vi "LabVIEW Verifier VI.vi"() -> ()   [LabVIEW 2020]
panel:
  out "Stabilization":u16(slide) scale=0.0..500.0
  out "Overall Verification":bool
  in  "Test Points & Results":T1(array[cluster])=[{"Volt Set Point (V)"=1.0, "Std Meas (V)"=0.0, "UUT Meas (V)"=0.0, "+/-Delta (V)"=0.1, "Result"=FALSE, "Error (mV)"=0.0}, {"Volt Set Point (V)"=3.3, "Std Meas (V)"=0.0, "UUT Meas (V)"=0.0, "+/-Delta (V)"=0.1, "Result"=FALSE, "Error (mV)"=0.0}, {"Volt Set Point (V)"=5.0, "Std Meas (V)"=0.0, "UUT Meas (V)"=0.0, "+/-Delta (V)"=0.1, "Result"=FALSE, "Error (mV)"=0.0}, {"Volt Set Point (V)"=10.0, "Std Meas (V)"=0.0, "UUT Meas (V)"=0.0, "+/-Delta (V)"=0.1, "Result"=FALSE, "Error (mV)"=0.0}, {"Volt Set Point (V)"=12.0, "Std Meas (V)"=0.0, "UUT Meas (V)"=0.0, "+/-Delta (V)"=0.1, "Result"=FALSE, "Error (mV)"=0.0}]
  # "Multimeter Calibration Verifier"
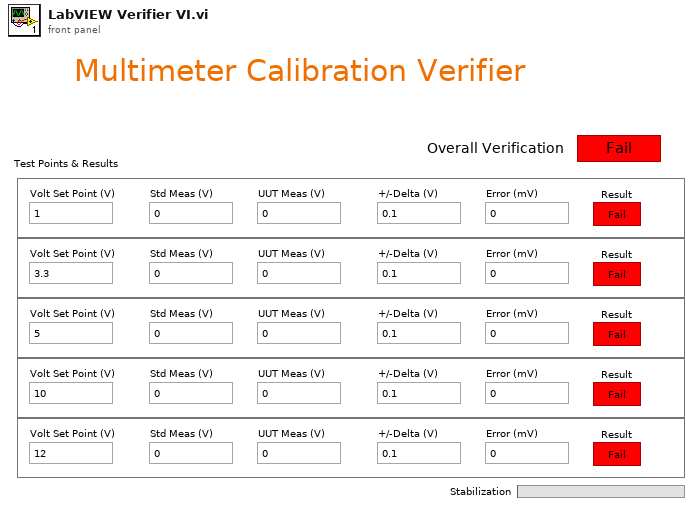
[diagram p1: front panel]
types:
  T1 = cluster{"Volt Set Point (V)":dbl, "Std Meas (V)":dbl, "UUT Meas (V)":dbl, "+/-Delta (V)":dbl, "Result":bool, "Error (mV)":dbl}[]
  T2 = cluster{"Volt Set Point (V)":dbl, "Std Meas (V)":dbl, "UUT Meas (V)":dbl, "+/-Delta (V)":dbl, "Result":bool, "Error (mV)":dbl}
  T3 = typedef "imagedata.ctl" = cluster{"image type":i32, "image depth":i32, "image":u8[], "mask":u8[], "colors":u32[], "Rectangle":cluster{"left":i16, "top":i16, "right":i16, "bottom":i16}}
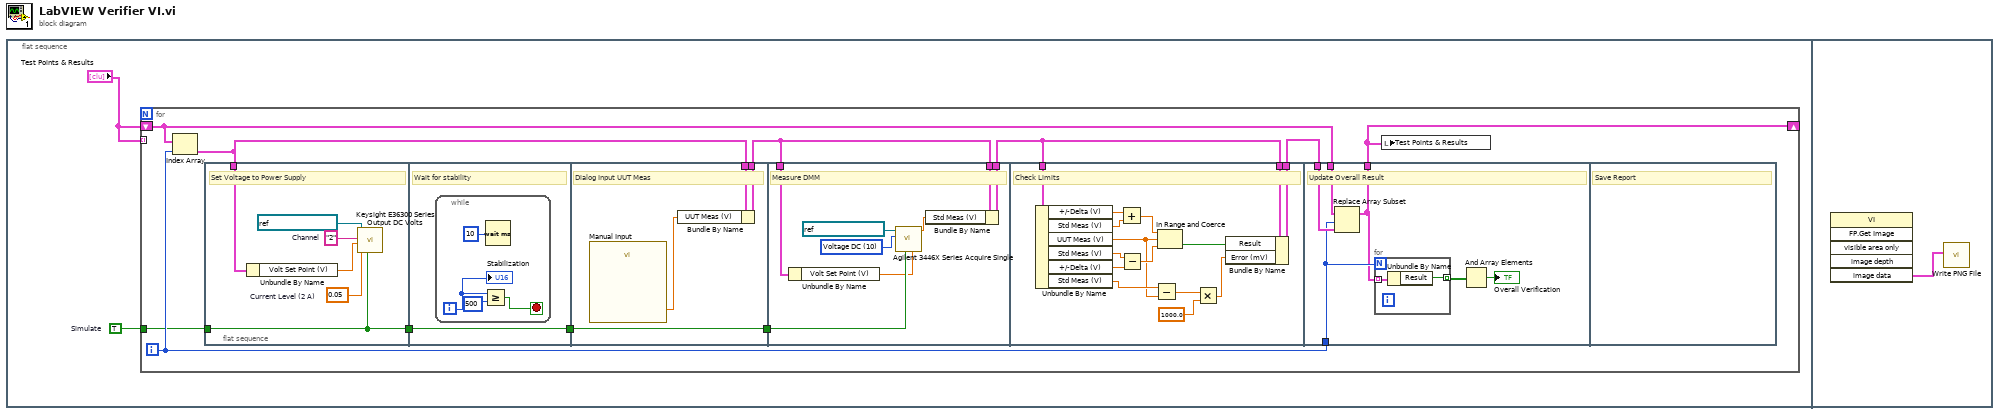
[diagram p0: block diagram]
diagram:
  n1 = flat-sequence {
    frame #0 {
      w1 = TRUE  # Simulate
      n2 = for {
        tunnel: "Test Points & Results" -> [_] mode=indexing
        shift-right: [w11] -> _
        shift-left: "Test Points & Results" -> [w10]
        tunnel: w1 -> [w7]
        i -> [w8]
        n3 = Index Array(array=w10, index=w8) -> (element=w9:T2)
        n4 = flat-sequence {
          tunnel: w9 -> [w19]
          tunnel: w7 -> [w14]
          tunnel: [w14] -> w6
          tunnel: w6 -> [w20]
          tunnel: [w20] -> w5
          tunnel: w9 -> [w28]
          tunnel: [w26] -> w3
          tunnel: w5 -> [w25]
          tunnel: [w25] -> w4
          tunnel: w3 -> [w34]
          tunnel: [w33] -> w13
          tunnel: w4 -> [w31]
          tunnel: w3 -> [w30]
          tunnel: w13 -> [w44]
          tunnel: w13 -> [w43]
          tunnel: [w42] -> w12
          tunnel: w10 -> [w57]
          tunnel: w8 -> [w53]
          tunnel: w12 -> [w56]
          tunnel: [w52] -> w11
          frame #0 {
            w15 = 0.05  # Current Level (2 A)
            w16 = "2"  # Channel
            # "Set Voltage to Power Supply"
            n5 = Unbundle By Name(w19) -> ("Volt Set Point (V)"=w18:dbl)
            n6 = call "Keysight E36300 Series Output DC Volts.vi"("Simulate"=w14, "Current Level (2 A)"=w15, "Voltage Level (1 V)"=w18, "Channel (1)"=w16, "VISA resource name"=refnum<visa-resource-name> "E36312A_PSU") -> ()  [unwired: 7 in]
          }
          frame #1 {
            # "Wait for stability"
            n7 = while {
              i -> [w23]
              stop <- w21 stop-if-true
              n8 = Greater Or Equal?(x=w23, y=500) -> (x >= y?=w21:bool)
              n9 = Wait (ms)(milliseconds to wait=u32 10) -> ()  [unwired: 1 out]
              "Stabilization" <- w23
            }
          }
          frame #2 {
            # "Dialog Input UUT Meas"
            n10 = call "Manual Input"() -> ("Voltage (V)"=w27:dbl)  [unwired: 17 in, 2 out]
            n11 = Bundle By Name(cluster=w28, "UUT Meas (V)"=w27) -> (w26:T2)
          }
          frame #3 {
            w35 = 10 items=["Continuity", "Current AC", "Current DC", "Diode", "Frequency", "Resistance 4-wire", "Period", "Resistance 2-wire", "Temperature", "Voltage AC", "Voltage DC", "Voltage DC Ratio", "Capacitance"] ("Measurement Function (10: Voltage DC)")
            # "Measure DMM"
            n12 = Unbundle By Name(w30) -> ("Volt Set Point (V)"=w29:dbl)
            n13 = call "Agilent 3446X Series Acquire Single.vi"("Sim. Volt Set Point (V)"=w29, "Simulate"=w31, "Measurement Function (10: Voltage DC)"=w35, "VISA resource name"=refnum<visa-resource-name> "34465A_DMM") -> ("Measurement"=w32:dbl)  [unwired: 7 in]
            n14 = Bundle By Name(cluster=w34, "Std Meas (V)"=w32) -> (w33:T2)
          }
          frame #4 {
            # "Check Limits"
            n15 = Unbundle By Name(w44) -> ("+/-Delta (V)"=w51:dbl, "Std Meas (V)"=w50:dbl, "UUT Meas (V)"=w39:dbl, "Std Meas (V)"=w48:dbl, "+/-Delta (V)"=w49:dbl, "Std Meas (V)"=w40:dbl)
            n16 = Add(x=w51, y=w50) -> (x+y=w47:dbl)
            n17 = Subtract(x=w48, y=w49) -> (x-y=w46:dbl)
            n18 = Subtract(x=w40, y=w39) -> (x-y=w38:dbl)
            n19 = In Range and Coerce(upper limit=w47, x=w39, lower limit=w46) -> (In Range?=w45:bool)  [unwired: 1 out]
            n20 = Multiply(x=w38, y=1000.0) -> (x*y=w37:dbl)
            n21 = Bundle By Name(cluster=w43, "Result"=w45, "Error (mV)"=w37) -> (w42:T2)
          }
          frame #5 {
            # "Update Overall Result"
            n22 = Replace Array Subset(array=w57, new element=w56, index=w53) -> (w52:T1)
            n23 = for {
              N: w53 -> [_]
              tunnel: w52 -> [w59] mode=indexing
              tunnel: [w58] -> w55 mode=indexing
              n24 = Unbundle By Name(w59) -> ("Result"=w58:bool)
            }
            n25 = And Array Elements(Boolean array=w55) -> (logical AND=→"Overall Verification":bool)
          }
          frame #6 {
            # "Save Report"
          }
        }
        n26 = local write "Test Points & Results"(w11) -> ()
      }
    }
    frame #1 {
      n27 = invoke class="VI" method="FP.Get Image"() -> ("image data"=w60:T3)  [unwired: 6 in, 5 out]
      n28 = call <vilib>:"Write PNG File.vi"("image data"=w60) -> ()  [unwired: 9 in, 2 out]
    }
  }
